vi "DiffDrivePoseEst2_New.vi"(4 "VisionMeasurementStdDevs":T2=[[0.1], [0.1], [0.05]], 6 "StateStdDevs":T2=[[0.02], [0.02], [0.01]], 7 "DIFF_DRIVE_KINEMATICS":T1 {"TrackWidth_Meters" format="%20.4f"}, 8 "InitialPose":T3={"TRANSLATION"={"X"=0.0, "Y"=0.0}, "ROTATION"={"VALUE"=0.0, "COS"=1.0, "SIN"=0.0}} {"ROTATION"."SIN" format="%13.4f"; "ROTATION"."COS" format="%13.4f"; "ROTATION"."VALUE" format="%13.4f"; "TRANSLATION"."Y" format="%14.3f"; "TRANSLATION"."X" format="%14.3f"}, 9 "RightDistance_M":dbl=0.02, 10 "LeftDistance_M":dbl=0.02, 11 "gyroAngle":T5={"VALUE"=0.0, "COS"=1.0, "SIN"=0.0} {"SIN" format="%13.4f"; "COS" format="%13.4f"; "VALUE" format="%13.4f"}) -> (0 "Error":errorcluster, 3 "DiffDrivePoseEstimate":T6={"M_Vision_K"=[], "m_nominal_dT"=0.0, "m_PrevTime_Sec"=0.0, "Pose_Buffer"={"TimeStamps"=[], "DataArray"=[], "Min_TimeStamp"=0.0, "Max_TimeStamp"=0.0, "ItemCount"=0, "MaxBufferTime"=0.0}, "Diff_Drive_Kinematics"={"TrackWidth_Meters"=0.0}, "Diff_Drive_Odom_2"={"M_POSE_Meters"={"TRANSLATION"={"X"=0.0, "Y"=0.0}, "ROTATION"={"VALUE"=0.0, "COS"=1.0, "SIN"=0.0}}, "M_GyroOffset"={"VALUE"=0.0, "COS"=1.0, "SIN"=0.0}, "M_PrevAngle"={"VALUE"=0.0, "COS"=1.0, "SIN"=0.0}, "M_PrevLeftDist_M"=0.0, "M_PrevRightDist_M"=0.0, "M_InitLeftDist_M"=0.0, "M_InitRightDist_M"=0.0}, "M_Q"=[[0.0], [0.0], [0.0]]} {"Diff_Drive_Odom_2"."M_PrevAngle"."SIN" format="%13.4f"; "Diff_Drive_Odom_2"."M_PrevAngle"."COS" format="%13.4f"; "Diff_Drive_Odom_2"."M_PrevAngle"."VALUE" format="%13.4f"; "Diff_Drive_Odom_2"."M_GyroOffset"."SIN" format="%13.4f"; "Diff_Drive_Odom_2"."M_GyroOffset"."COS" format="%13.4f"; "Diff_Drive_Odom_2"."M_GyroOffset"."VALUE" format="%13.4f"; "Diff_Drive_Odom_2"."M_POSE_Meters"."ROTATION"."SIN" format="%13.4f"; "Diff_Drive_Odom_2"."M_POSE_Meters"."ROTATION"."COS" format="%13.4f"; "Diff_Drive_Odom_2"."M_POSE_Meters"."ROTATION"."VALUE" format="%13.4f"; "Diff_Drive_Odom_2"."M_POSE_Meters"."TRANSLATION"."Y" format="%14.3f"; "Diff_Drive_Odom_2"."M_POSE_Meters"."TRANSLATION"."X" format="%14.3f"; "Diff_Drive_Kinematics"."TrackWidth_Meters" format="%20.4f"})   [LabVIEW 2019, in "Trajectory_Library.lvlib"]
doc: "This class wraps Differential Drive Odometry to fuse latency-compensated vision measurements with differential drive encoder measurements. It is intended to be a drop-in replacement for DiffDrvOdom2; in fact, if you never call DiffDrvPoseEst2_AddVisionMeasurement and only call DiffDrvPoseEst2_Update then this will behave exactly the same as DiffDrvOdom2.\n \nDiffDrvPoseEst2_Update should be called every robot loop.\n \nDiffDrvPoseEst2_AddVisionMeasurement can be called as infrequently as you want. If you never call it then this set of VI will behave exactly like regular encoder odometry.\n\nConstructs a DifferentialDrivePoseEstimator.\n\nThe default standard deviations of the model states are 0.02 meters for x, 0.02 meters for y, and 0.01 radians for heading. The default standard deviations of the vision measurements are 0.1 meters for x, 0.1 meters for y, and 0.1 radians for heading.\n\nInputs: \n - kinematics -- DiffDriveKinematics -- A correctly-configured kinematics data cluster for your drivetrain.\n - gyroAngle -- Rotation2d -- The current gyro angle.\n - leftDistanceMeters -- double -- The distance traveled by the left encoder.\n - rightDistanceMeters -- double -- The distance traveled by the right encoder.\n - initialPoseMeters -- Pose2d -- The starting pose estimate.\n - stateStdDevs -- <3,1> matrix -- Standard deviations of the pose estimate (x position in meters, y position in meters, and heading in radians). Increase these numbers to trust your state estimate less.\n - visionMeasurementStdDevs -- <3,1> matrix -- Standard deviations of the vision pose measurement (x position in meters, y position in meters, and heading in radians). Increase these numbers to trust the vision pose measurement less.\n \nOutputs:\n -- DiffDrivePoseEst2 -- DiffDrivePoseEst2 -- Created data cluster."
uses:
  Trajectory_Library.lvlib
  TypeDef/DIFF_DRIVE_POSE_EST2.ctl
  <vilib>/Analysis/Matrix/Datatypes/RealMatrix.ctl
  TypeDef/TIME_INTERPOLATABLE_VARIANT.ctl
  TypeDef/DIFF_DRIVE_KINEMATICS.ctl
  TypeDef/DIFF_DRIVE_ODOM2.ctl
  TypeDef/POSE2D.ctl
  TypeDef/TRANSLATION2D.ctl
  TypeDef/ROTATION2D.ctl
  MatBuilder_Create.vi
  <vilib>/Rock Robotics/SystemInterfaces/NetworkCommunication/NetComm_UsageReport_report.vi
  Pose2d_getRotation.vi
  Rotation2d_Minus.vi
  Rotation2d_UnaryMinus.vi
  Rotation2d_RotateBy.vi
  Rotation2d_CreateAngle.vi
  Rotation2d_CreateXY.vi
  Util_CalcDist.vi
  Globals/Util_LibraryGlobals.vi
  <vilib>/Analysis/Matrix/NI_Matrix.lvlib
panel:
  # "<3,1>"
  # "<3, 1>"
  # "<3, 1>"
  # "<3, 3>"
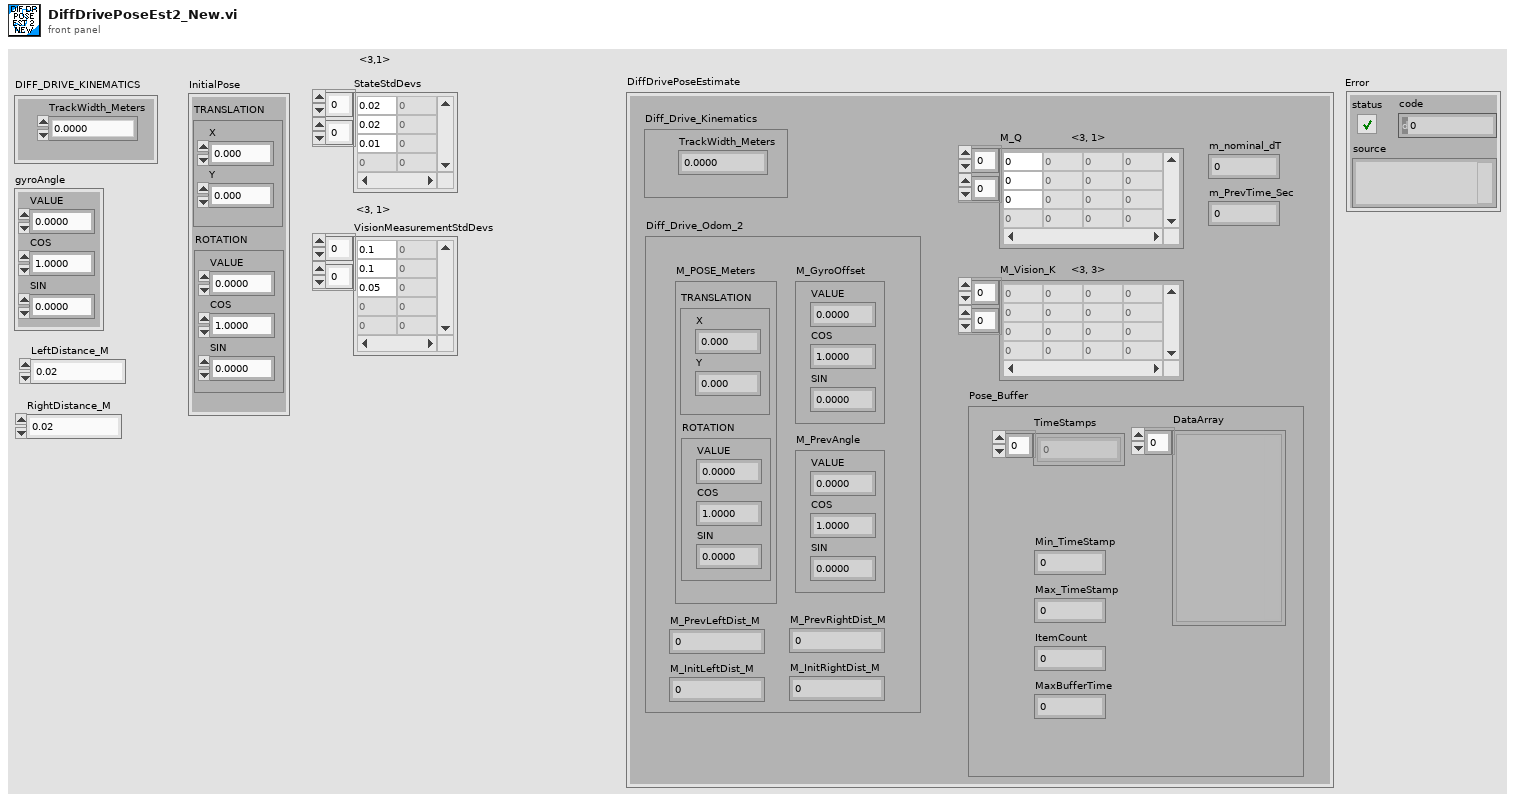
[diagram p1: front panel]
types:
  T1 = typedef "Trajectory_Library.lvlib/DIFF_DRIVE_KINEMATICS.ctl" = cluster{"TrackWidth_Meters":dbl}
  T2 = typedef "NI_Matrix.lvlib/RealMatrix.ctl" = dbl[][]
  T3 = typedef "Trajectory_Library.lvlib/POSE2D.ctl" = cluster{"TRANSLATION":T4, "ROTATION":T5}
  T4 = typedef "Trajectory_Library.lvlib/TRANSLATION2D.ctl" = cluster{"X":dbl, "Y":dbl}
  T5 = typedef "Trajectory_Library.lvlib/ROTATION2D.ctl" = cluster{"VALUE":dbl, "COS":dbl, "SIN":dbl}
  T6 = typedef "Trajectory_Library.lvlib/DIFF_DRIVE_POSE_EST2.ctl" = cluster{"M_Vision_K":T2, "m_nominal_dT":dbl, "m_PrevTime_Sec":dbl, "Pose_Buffer":T7, "Diff_Drive_Kinematics":T1, "Diff_Drive_Odom_2":T8, "M_Q":T2}
  T7 = typedef "Trajectory_Library.lvlib/TIME_INTERPOLATABLE_VARIANT.ctl" = cluster{"TimeStamps":dbl[], "DataArray":variant[], "Min_TimeStamp":dbl, "Max_TimeStamp":dbl, "ItemCount":i32, "MaxBufferTime":dbl}
  T8 = typedef "Trajectory_Library.lvlib/DIFF_DRIVE_ODOM2.ctl" = cluster{"M_POSE_Meters":T3, "M_GyroOffset":T5, "M_PrevAngle":T5, "M_PrevLeftDist_M":dbl, "M_PrevRightDist_M":dbl, "M_InitLeftDist_M":dbl, "M_InitRightDist_M":dbl}
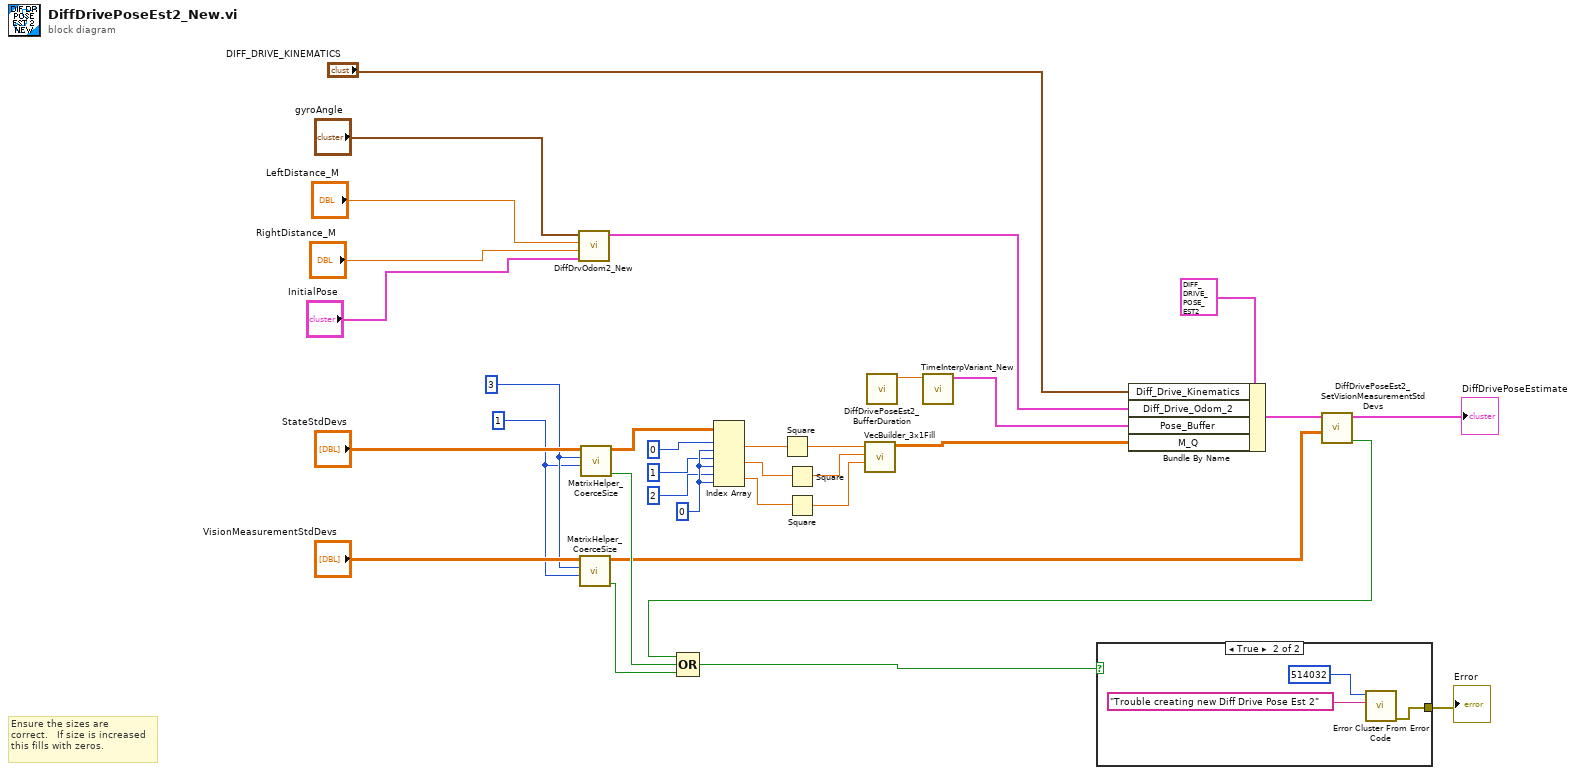
[diagram p0: block diagram]
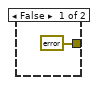
[diagram p2: hidden frame]
diagram:
  w17 = 0 ("index (col)")
  w20 = 1 ("Outputs")
  w21 = 3 ("States")
  # "Ensure the sizes are\ncorrect.   If size is increased \nthis fills with zeros."
  n1 = call "DiffDrvOdom2_New.vi"("Initial Pose Meters"="InitialPose", "Initial Right Distance M"="RightDistance_M", "Initial Left Distance M"="LeftDistance_M", "Initial Gyro Reading"="gyroAngle") -> ("Out DIFF_DRIVE_ODOM"=w23:T8)  [unwired: 7 in]
  n2 = call "MatrixHelper_CoerceSize.vi"("Columns"=w20, "Rows"=w21, "input matrix"="VisionMeasurementStdDevs") -> ("Coerced"=w7:bool, "output matrix"=w2:T2)  [unwired: 7 in]
  n3 = call "MatrixHelper_CoerceSize.vi"("Columns"=w20, "Rows"=w21, "input matrix"="StateStdDevs") -> ("Coerced"=w31:bool, "output matrix"=w19:T2)  [unwired: 7 in]
  n4 = Index Array(array=w19, index (row) #1=0 ("index (row)"), index (col) #1=w17, index (row) #2=1 ("index (row)"), index (col) #2=w17, index (row) #3=2 ("index (row)"), index (col) #3=w17) -> (element #1=w14:dbl, element #2=w13:dbl, element #3=w12:dbl)
  n5 = Square(x=w14) -> (x^2=w11:dbl)
  n6 = Square(x=w13) -> (x^2=w10:dbl)
  n7 = Square(x=w12) -> (x^2=w9:dbl)
  n8 = call "VecBuilder_3x1Fill.vi"("R2"=w9, "R1"=w10, "R0"=w11) -> ("output matrix"=w8:T2)  [unwired: 8 in]
  n9 = call "DiffDrivePoseEst2_BufferDuration.vi"() -> ("Buffer Duration (Sec)"=w1:dbl)  [unwired: 11 in]
  n10 = call "TimeInterpVariant_New.vi"("MaxTime"=w1) -> ("TimeInterpVariant"=w22:T7)  [unwired: 10 in]
  n11 = Bundle By Name(cluster=T6 {"M_Vision_K"=[], "m_nominal_dT"=0.0, "m_PrevTime_Sec"=0.0, "Pose_Buffer"={"TimeStamps"=[], "DataArray"=[], "Min_TimeStamp"=0.0, "Max_TimeStamp"=0.0, "ItemCount"=0, "MaxBufferTime"=0.0}, "Diff_Drive_Kinematics"={"TrackWidth_Meters"=0.0}, "Diff_Drive_Odom_2"={"M_POSE_Meters"={"TRANSLATION"={"X"=0.0, "Y"=0.0}, "ROTATION"={"VALUE"=0.0, "COS"=1.0, "SIN"=0.0}}, "M_GyroOffset"={"VALUE"=0.0, "COS"=1.0, "SIN"=0.0}, "M_PrevAngle"={"VALUE"=0.0, "COS"=1.0, "SIN"=0.0}, "M_PrevLeftDist_M"=0.0, "M_PrevRightDist_M"=0.0, "M_InitLeftDist_M"=0.0, "M_InitRightDist_M"=0.0}, "M_Q"=[[0.0], [0.0], [0.0]]} ("DiffDrivePoseEstimate 2"), "Diff_Drive_Kinematics"="DIFF_DRIVE_KINEMATICS", "Diff_Drive_Odom_2"=w23, "Pose_Buffer"=w22, "M_Q"=w8) -> (w5:T6)
  n12 = call "DiffDrivePoseEst2_SetVisionMeasurementStdDevs.vi"("VisionMeasurementStdDevs"=w2, "in DiffDrivePoseEstimate2"=w5) -> ("Size Coerced"=w3:bool, "Out DiffDrivePoseEstimate2"=→"DiffDrivePoseEstimate":T6)  [unwired: 8 in]
  n13 = Compound Arithmetic op=OR(w3, w31, w7) -> (w6:bool)
  n14 = case shown="True" w6 {
    tunnel: [errorcluster {"status"=FALSE, "code"=0, "source"=""} ("error out") w37] -> w30
    frame False {
    }
    frame True {
      n15 = call <vilib>:"Error Cluster From Error Code.vi"("error message (\"\")"="Trouble creating new Diff Drive Pose Est 2" ("error message (\"\")"), "error code (0)"=514032) -> ("error out"=w37:errorcluster)  [unwired: 7 in]
    }
  }
  "Error" <- w30
